vi "Request Message Control Label.vi"() -> (0 "Messages References Control Label":string)   [LabVIEW 2018, in "Scripting.lvlib"]
uses:
  Scripting.lvlib
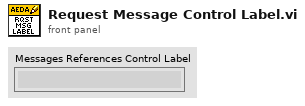
[diagram p1: front panel]
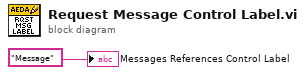
[diagram p0: block diagram]
diagram:
  "Messages References Control Label" <- "Message" ("y")
